vi "File - Save Controls to INI.vi"(7 "Section":string, 8 "error in (no error)":errorcluster, 9 "Array of References":refnum<vi>[](array[refnum]), 11 "INI File":path) -> (0 "error out":errorcluster)   [LabVIEW 2020]
doc: "Saves the values of a group of controls (passed as an array of references) to an INI file.\n\nThe control names are used for the key names (with spaces removed).\n\nWorks with digital/boolean/string/path/VISAResourceName and single level clusters."
uses:
  <vilib>/Utility/config.llb/Write Key (Double).vi
  <vilib>/Utility/config.llb/Write Key (String).vi
  <vilib>/Utility/config.llb/NI_LVConfig.lvlib
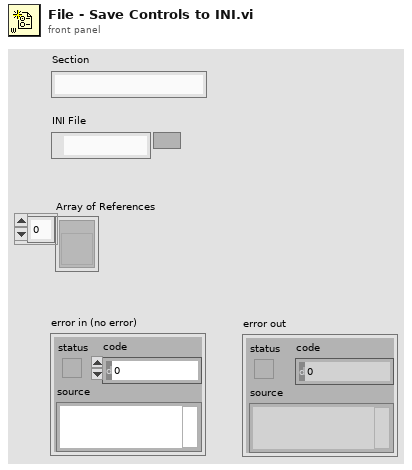
[diagram p1: front panel]
types:
  T1 = typedef "NI_LVConfig.lvlib/Config Data RefNum.ctl" = refnum<k1>
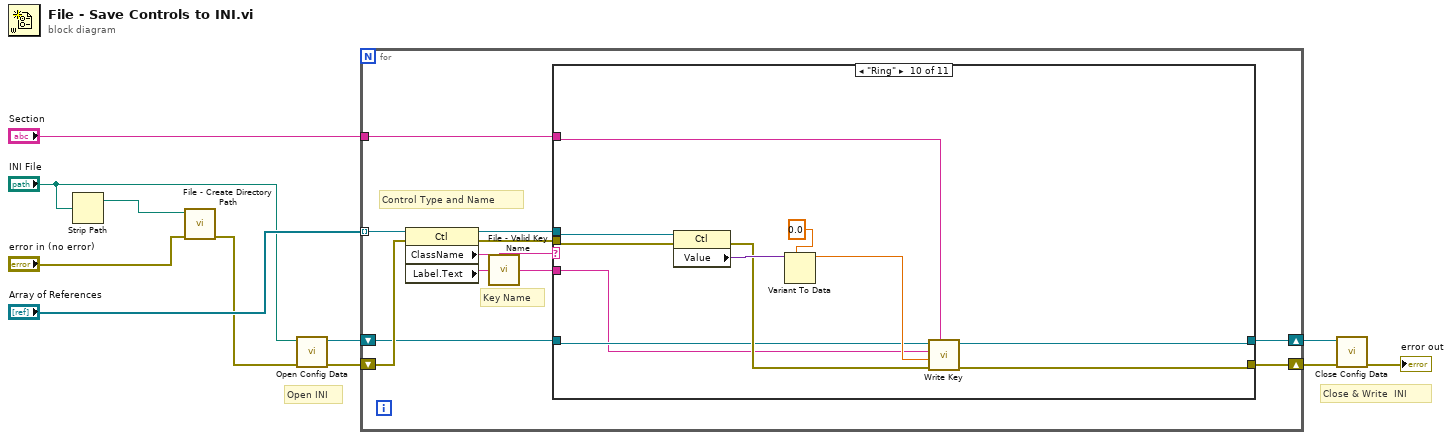
[diagram p0: block diagram]
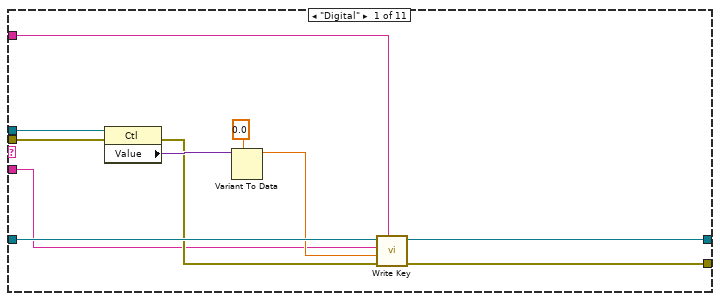
[diagram p2: hidden frame]
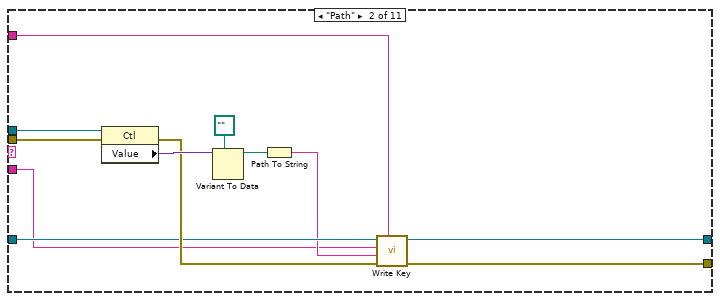
[diagram p3: hidden frame]
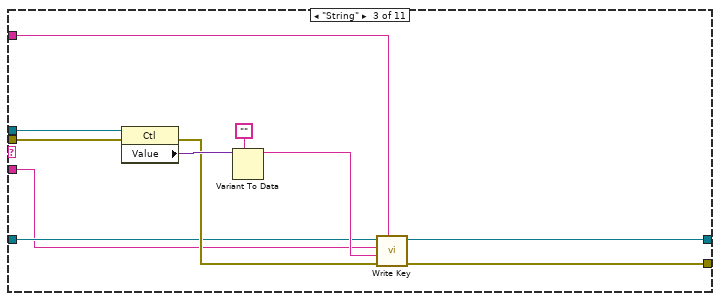
[diagram p4: hidden frame]
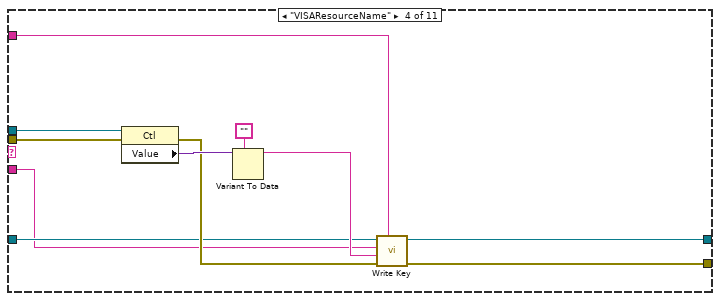
[diagram p5: hidden frame]
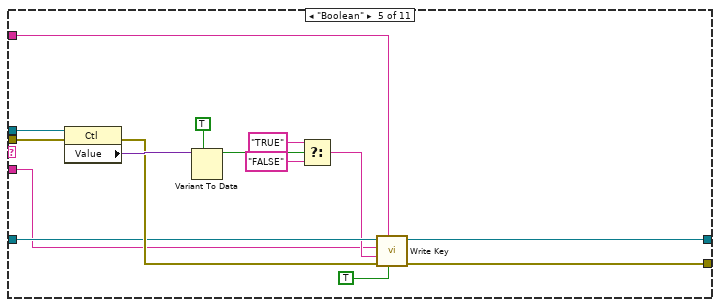
[diagram p6: hidden frame]
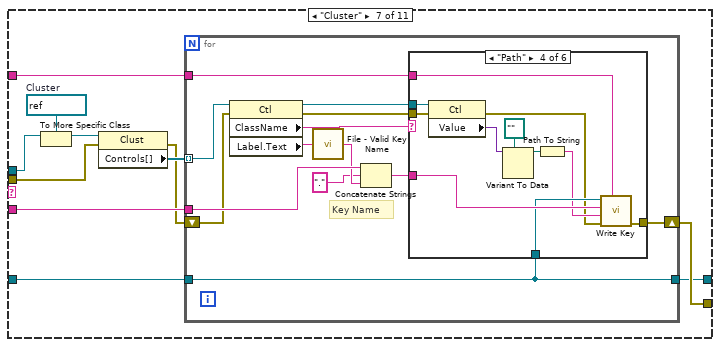
[diagram p8: hidden frame]
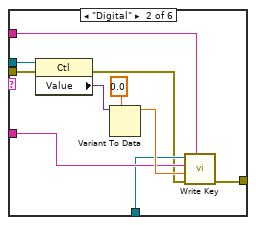
[diagram p10: hidden frame]
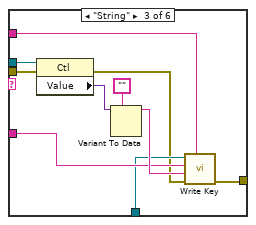
[diagram p11: hidden frame]
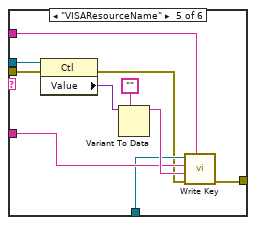
[diagram p12: hidden frame]
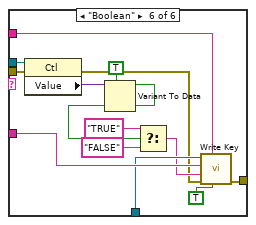
[diagram p13: hidden frame]
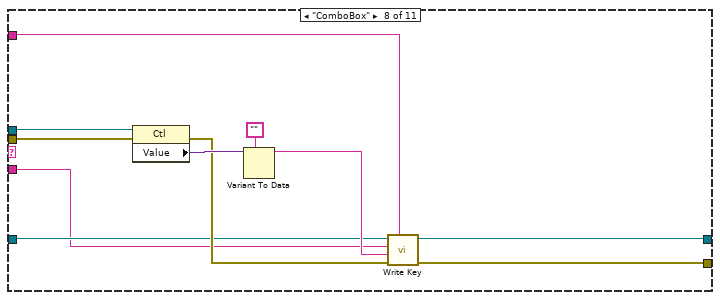
[diagram p14: hidden frame]
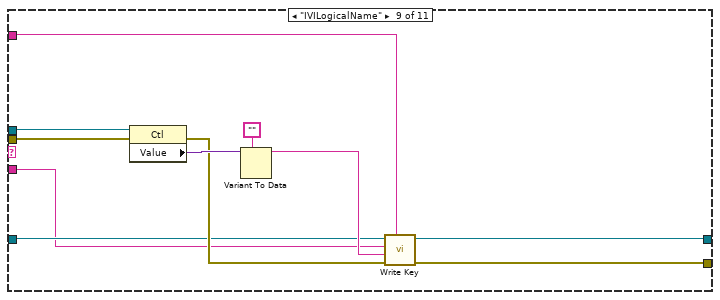
[diagram p15: hidden frame]
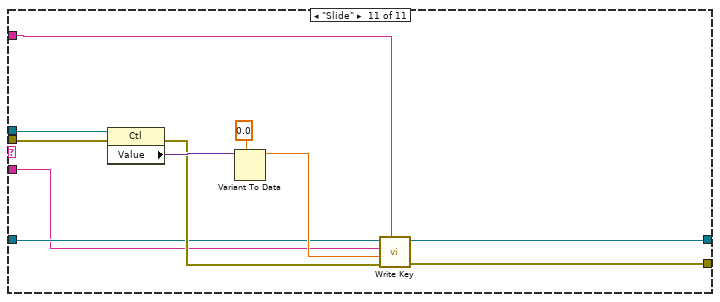
[diagram p16: hidden frame]
diagram:
  # "Close & Write  INI"
  # "Open INI"
  n1 = Strip Path(path="INI File") -> (stripped path=w8:path)  [unwired: 1 out]
  n2 = call "File - Create Directory Path.vi"("error in (no error)"="error in (no error)", "Path"=w8) -> ("error out"=w6:errorcluster)  [unwired: 8 in, 1 out]
  n3 = call <vilib>:"Open Config Data.vi"("error in (no error)"=w6, "configuration file path"="INI File") -> ("error out"=w5:errorcluster, "refnum"=w3:T1)  [unwired: 7 in, 1 out]
  n4 = for {
    tunnel: "Array of References" -> [w22] mode=indexing
    tunnel: "Section" -> [w19]
    shift-right: [w18] -> w9
    shift-left: w5 -> [w17]
    shift-right: [w15] -> w1
    shift-left: w3 -> [w14]
    # "Key Name"
    # "Control Type and Name"
    n5 = property class="Ctl"(reference=w22, error in=w17) -> (reference out=w20:refnum<vi>, error out=w16:errorcluster, "ClassName"=w21:string, "Label.Text"=w13:string)
    n6 = call "File - Valid Key Name.vi"("Key Name In"=w13) -> ("Key Name Out"=w12:string)  [unwired: 4 in]
    n7 = case shown="\"Ring\"" w21 {
      tunnel: w20 -> [w33 w45 w56 w67 w82 _ w95 w170 w181 w193 w203]
      tunnel: w12 -> [w23 w34 w46 w57 w69 _ w90 w167 w178 w188 w200]
      tunnel: w19 -> [w29 w41 w52 w63 w75 _ w88 w171 w182 w194 w204]
      tunnel: w16 -> [w30 w42 w53 w64 w76 w84 w91 w169 w180 w192 w202]
      tunnel: [w26 w40 w51 w62 w68 w84 w89 w165 w176 w189 w198] -> w18
      tunnel: [w27 w37 w48 w59 w73 w83 w86 w166 w177 w190 w199] -> w15
      tunnel: w14 -> [w28 w38 w47 w58 w72 w83 w87 w168 w179 w191 w201]
      frame "Digital" {
        n8 = property class="Ctl"(reference=w33, error in=w30) -> (error out=w25:errorcluster, "Value"=w32:variant)  [unwired: 1 out]
        n9 = Variant To Data(type=0.0 ("Total"), Variant=w32) -> (data=w24:dbl)  [unwired: 1 in, 1 out]
        n10 = call-poly <vilib>:"Write Key.vi"("section"=w29, "error in (no error)"=w25, "value"=w24, "key"=w23, "refnum"=w28) -> ("error out"=w26:errorcluster, "refnum out"=w27:T1)  [unwired: 4 in, 1 out]
      }
      frame "Path" {
        n11 = property class="Ctl"(reference=w45, error in=w42) -> (error out=w39:errorcluster, "Value"=w44:variant)  [unwired: 1 out]
        n12 = Variant To Data(type=path "", Variant=w44) -> (data=w36:path)  [unwired: 1 in, 1 out]
        n13 = Path To String(path=w36) -> (string=w35:string)
        n14 = call-poly <vilib>:"Write Key.vi"("section"=w41, "error in (no error)"=w39, "value"=w35, "key"=w34, "refnum"=w38) -> ("error out"=w40:errorcluster, "refnum out"=w37:T1)  [unwired: 4 in, 1 out]
      }
      frame "String" {
        n15 = property class="Ctl"(reference=w56, error in=w53) -> (error out=w50:errorcluster, "Value"=w55:variant)  [unwired: 1 out]
        n16 = Variant To Data(type="", Variant=w55) -> (data=w49:string)  [unwired: 1 in, 1 out]
        n17 = call-poly <vilib>:"Write Key.vi"("section"=w52, "error in (no error)"=w50, "value"=w49, "key"=w46, "refnum"=w47) -> ("error out"=w51:errorcluster, "refnum out"=w48:T1)  [unwired: 4 in, 1 out]
      }
      frame "VISAResourceName" {
        n18 = property class="Ctl"(reference=w67, error in=w64) -> (error out=w61:errorcluster, "Value"=w66:variant)  [unwired: 1 out]
        n19 = Variant To Data(type="", Variant=w66) -> (data=w60:string)  [unwired: 1 in, 1 out]
        n20 = call-poly <vilib>:"Write Key.vi"("section"=w63, "error in (no error)"=w61, "value"=w60, "key"=w57, "refnum"=w58) -> ("error out"=w62:errorcluster, "refnum out"=w59:T1)  [unwired: 4 in, 1 out]
      }
      frame "Boolean" {
        n21 = property class="Ctl"(reference=w82, error in=w76) -> (error out=w74:errorcluster, "Value"=w81:variant)  [unwired: 1 out]
        n22 = Variant To Data(type=TRUE, Variant=w81) -> (data=w79:bool)  [unwired: 1 in, 1 out]
        n23 = Select(t="TRUE", s=w79, f="FALSE") -> (s? t:f=w71:string)
        n24 = call-poly <vilib>:"Write Key.vi"("write raw string? (F)"=TRUE, "section"=w75, "error in (no error)"=w74, "value"=w71, "key"=w69, "refnum"=w72) -> ("error out"=w68:errorcluster, "refnum out"=w73:T1)  [unwired: 3 in, 1 out]
      }
      frame Default {
      }
      frame "Cluster" {
        w93 = refnum<vi> refnum  # Cluster
        n25 = To More Specific Class(target class=w93, reference=w95) -> (specific class reference=w94:refnum<vi>)  [unwired: 1 in, 1 out]
        n26 = property class="Clust"(reference=w94, error in=w91) -> (error out=w85:errorcluster, "Controls[]"=w92:refnum<vi>[])  [unwired: 1 out]
        n27 = for {
          tunnel: w92 -> [w108] mode=indexing
          tunnel: w90 -> [w105]
          shift-right: [w101] -> w89
          shift-left: w85 -> [w97]
          tunnel: w88 -> [w99]
          tunnel: w87 -> [w98]
          tunnel: [w98] -> w86
          # "Key Name"
          n28 = property class="Ctl"(reference=w108, error in=w97) -> (reference out=w100:refnum<vi>, error out=w96:errorcluster, "ClassName"=w106:string, "Label.Text"=w107:string)
          n29 = call "File - Valid Key Name.vi"("Key Name In"=w107) -> ("Key Name Out"=w104:string)  [unwired: 4 in]
          n30 = Concatenate Strings(w105, ".", w104) -> (w102:string)
          n31 = case shown="\"Path\"" w106 {
            tunnel: w102 -> [_ w113 w123 w134 w144 w159]
            tunnel: [w109 w116 w126 w137 w147 w161] -> w101
            tunnel: w100 -> [_ w119 w129 w140 w150 w164]
            tunnel: w99 -> [_ w115 w125 w136 w146 w160]
            tunnel: w98 -> [_ w112 w122 w133 w143 w158]
            tunnel: w96 -> [w109 w111 w121 w131 w142 w152]
            frame Default {
            }
            frame "Digital" {
              n32 = property class="Ctl"(reference=w119, error in=w111) -> (error out=w110:errorcluster, "Value"=w117:variant)  [unwired: 1 out]
              n33 = Variant To Data(type=0.0 ("Total"), Variant=w117) -> (data=w114:dbl)  [unwired: 1 in, 1 out]
              n34 = call-poly <vilib>:"Write Key.vi"("section"=w115, "error in (no error)"=w110, "value"=w114, "key"=w113, "refnum"=w112) -> ("error out"=w116:errorcluster)  [unwired: 4 in, 2 out]
            }
            frame "String" {
              n35 = property class="Ctl"(reference=w129, error in=w121) -> (error out=w120:errorcluster, "Value"=w127:variant)  [unwired: 1 out]
              n36 = Variant To Data(type="" ("Total"), Variant=w127) -> (data=w124:string)  [unwired: 1 in, 1 out]
              n37 = call-poly <vilib>:"Write Key.vi"("section"=w125, "error in (no error)"=w120, "value"=w124, "key"=w123, "refnum"=w122) -> ("error out"=w126:errorcluster)  [unwired: 4 in, 2 out]
            }
            frame "Path" {
              n38 = property class="Ctl"(reference=w140, error in=w131) -> (error out=w130:errorcluster, "Value"=w138:variant)  [unwired: 1 out]
              n39 = Variant To Data(type=path "" ("Total"), Variant=w138) -> (data=w135:path)  [unwired: 1 in, 1 out]
              n40 = Path To String(path=w135) -> (string=w132:string)
              n41 = call-poly <vilib>:"Write Key.vi"("section"=w136, "error in (no error)"=w130, "value"=w132, "key"=w134, "refnum"=w133) -> ("error out"=w137:errorcluster)  [unwired: 4 in, 2 out]
            }
            frame "VISAResourceName" {
              n42 = property class="Ctl"(reference=w150, error in=w142) -> (error out=w141:errorcluster, "Value"=w148:variant)  [unwired: 1 out]
              n43 = Variant To Data(type="" ("Total"), Variant=w148) -> (data=w145:string)  [unwired: 1 in, 1 out]
              n44 = call-poly <vilib>:"Write Key.vi"("section"=w146, "error in (no error)"=w141, "value"=w145, "key"=w144, "refnum"=w143) -> ("error out"=w147:errorcluster)  [unwired: 4 in, 2 out]
            }
            frame "Boolean" {
              n45 = property class="Ctl"(reference=w164, error in=w152) -> (error out=w151:errorcluster, "Value"=w162:variant)  [unwired: 1 out]
              n46 = Variant To Data(type=TRUE, Variant=w162) -> (data=w155:bool)  [unwired: 1 in, 1 out]
              n47 = Select(t="TRUE", s=w155, f="FALSE") -> (s? t:f=w154:string)
              n48 = call-poly <vilib>:"Write Key.vi"("write raw string? (F)"=TRUE, "section"=w160, "error in (no error)"=w151, "value"=w154, "key"=w159, "refnum"=w158) -> ("error out"=w161:errorcluster)  [unwired: 3 in, 2 out]
            }
          }
        }
      }
      frame "ComboBox" {
        n49 = property class="Ctl"(reference=w170, error in=w169) -> (error out=w173:errorcluster, "Value"=w175:variant)  [unwired: 1 out]
        n50 = Variant To Data(type="", Variant=w175) -> (data=w172:string)  [unwired: 1 in, 1 out]
        n51 = call-poly <vilib>:"Write Key.vi"("section"=w171, "error in (no error)"=w173, "value"=w172, "key"=w167, "refnum"=w168) -> ("error out"=w165:errorcluster, "refnum out"=w166:T1)  [unwired: 4 in, 1 out]
      }
      frame "IVILogicalName" {
        n52 = property class="Ctl"(reference=w181, error in=w180) -> (error out=w184:errorcluster, "Value"=w186:variant)  [unwired: 1 out]
        n53 = Variant To Data(type="", Variant=w186) -> (data=w183:string)  [unwired: 1 in, 1 out]
        n54 = call-poly <vilib>:"Write Key.vi"("section"=w182, "error in (no error)"=w184, "value"=w183, "key"=w178, "refnum"=w179) -> ("error out"=w176:errorcluster, "refnum out"=w177:T1)  [unwired: 4 in, 1 out]
      }
      frame "Ring" {
        n55 = property class="Ctl"(reference=w193, error in=w192) -> (error out=w196:errorcluster, "Value"=w197:variant)  [unwired: 1 out]
        n56 = Variant To Data(type=0.0 ("Total"), Variant=w197) -> (data=w195:dbl)  [unwired: 1 in, 1 out]
        n57 = call-poly <vilib>:"Write Key.vi"("section"=w194, "error in (no error)"=w196, "value"=w195, "key"=w188, "refnum"=w191) -> ("error out"=w189:errorcluster, "refnum out"=w190:T1)  [unwired: 4 in, 1 out]
      }
      frame "Slide" {
        n58 = property class="Ctl"(reference=w203, error in=w202) -> (error out=w206:errorcluster, "Value"=w208:variant)  [unwired: 1 out]
        n59 = Variant To Data(type=0.0 ("Total"), Variant=w208) -> (data=w205:dbl)  [unwired: 1 in, 1 out]
        n60 = call-poly <vilib>:"Write Key.vi"("section"=w204, "error in (no error)"=w206, "value"=w205, "key"=w200, "refnum"=w201) -> ("error out"=w198:errorcluster, "refnum out"=w199:T1)  [unwired: 4 in, 1 out]
      }
    }
  }
  n61 = call <vilib>:"Close Config Data.vi"("error in (no error)"=w9, "refnum"=w1) -> ("error out"=→"error out":errorcluster)  [unwired: 8 in, 1 out]
